vi "Actual Corrected Flow SI.vi"(8 "Error In":errorcluster, 10 "Channel (0)":i32, 11 "VISA resource name":refnum<visa-resource-name>) -> (0 "Error Out":errorcluster, 1 "Corrected Gas Flow":dbl[unit], 3 "dup VISA resource name":refnum<visa-resource-name>)   [LabVIEW 2011, in "MGC647C.lvlib"]
doc: "Read actual gas flow with respect to gas correction factor."
uses:
  <instrlib>/MGC647C/MGC647C.lvlib
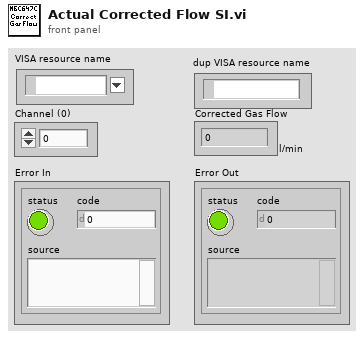
[diagram p1: front panel]
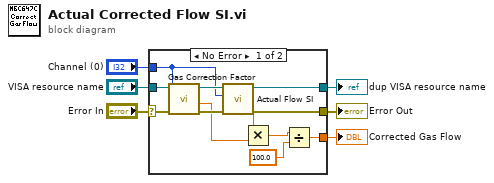
[diagram p0: block diagram]
diagram:
  n1 = case shown="No Error" "Error In" {
    selector: "Error In" -> [w10 w19]
    tunnel: "VISA resource name" -> [w18 w20]
    tunnel: "Channel (0)" -> [w15 _]
    tunnel: [w13 _] -> w4
    tunnel: [w12 w20] -> w3
    tunnel: [w11 w19] -> w2
    frame No Error {
      n2 = call <instrlib>:"Gas Correction Factor.vi"("Error In"=w10, "Channel (0)"=w15, "VISA resource name"=w18) -> ("Error Out"=w16:errorcluster, "Gas Correction Factor out"=w8:dbl, "dup VISA resource name"=w17:refnum<visa-resource-name>)  [unwired: 6 in]
      n3 = call <instrlib>:"Actual Flow SI.vi"("Error In"=w16, "Channel (0)"=w15, "VISA resource name"=w17) -> ("Error Out"=w11:errorcluster, "Flow"=w9:dbl[unit], "dup VISA resource name"=w12:refnum<visa-resource-name>)  [unwired: 6 in]
      n4 = Multiply(x=w9, y=w8) -> (x*y=w7:dbl[unit])
      n5 = Divide(x=w7, y=100.0) -> (x/y=w13:dbl[unit])
    }
    frame Error {
    }
  }
  "Corrected Gas Flow" <- w4
  "dup VISA resource name" <- w3
  "Error Out" <- w2
